vi "Splitting_without_Origin_Solution-1.vi"(6 "[IN] Crossconn\nection corrected":bool, 8 "error IN":errorcluster, 9 "[IN] # of Track with\nFirst Problem Point":i32, 10 "[IN] Index of First Pro\nblem Point Inside Track":i32, 11 "[IN] Still connected\ntracks in group":T2) -> (0 "error OUT":errorcluster, 3 "[OUT] Clusters for Re\nconstructed Tracks":T1, 4 "[OUT] Problem with 11 Point\nwithout Origin Resolved":bool)   [LabVIEW 2013]
doc: "Suprogram resolves the problem of splitting with no origin: \n- if further points don't merge again (assumption that they aren't equaul to \"101\" or \"111\") \n - then splitting points just loose their problem status and become origins for two different tracks"
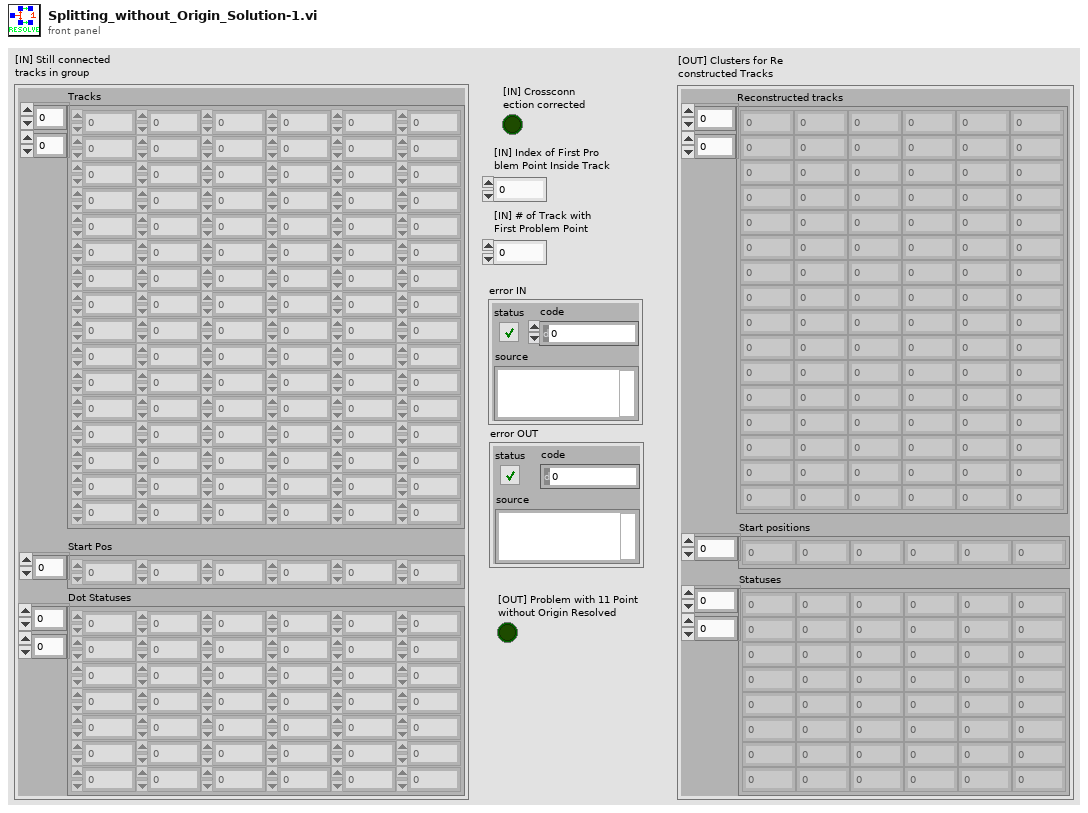
[diagram p1: front panel]
types:
  T1 = cluster{"Reconstructed tracks":dbl[][], "Start positions":i32[], "Statuses":i16[][]}
  T2 = cluster{"Tracks":dbl[][], "Start Pos":i32[], "Dot Statuses":i16[][]}
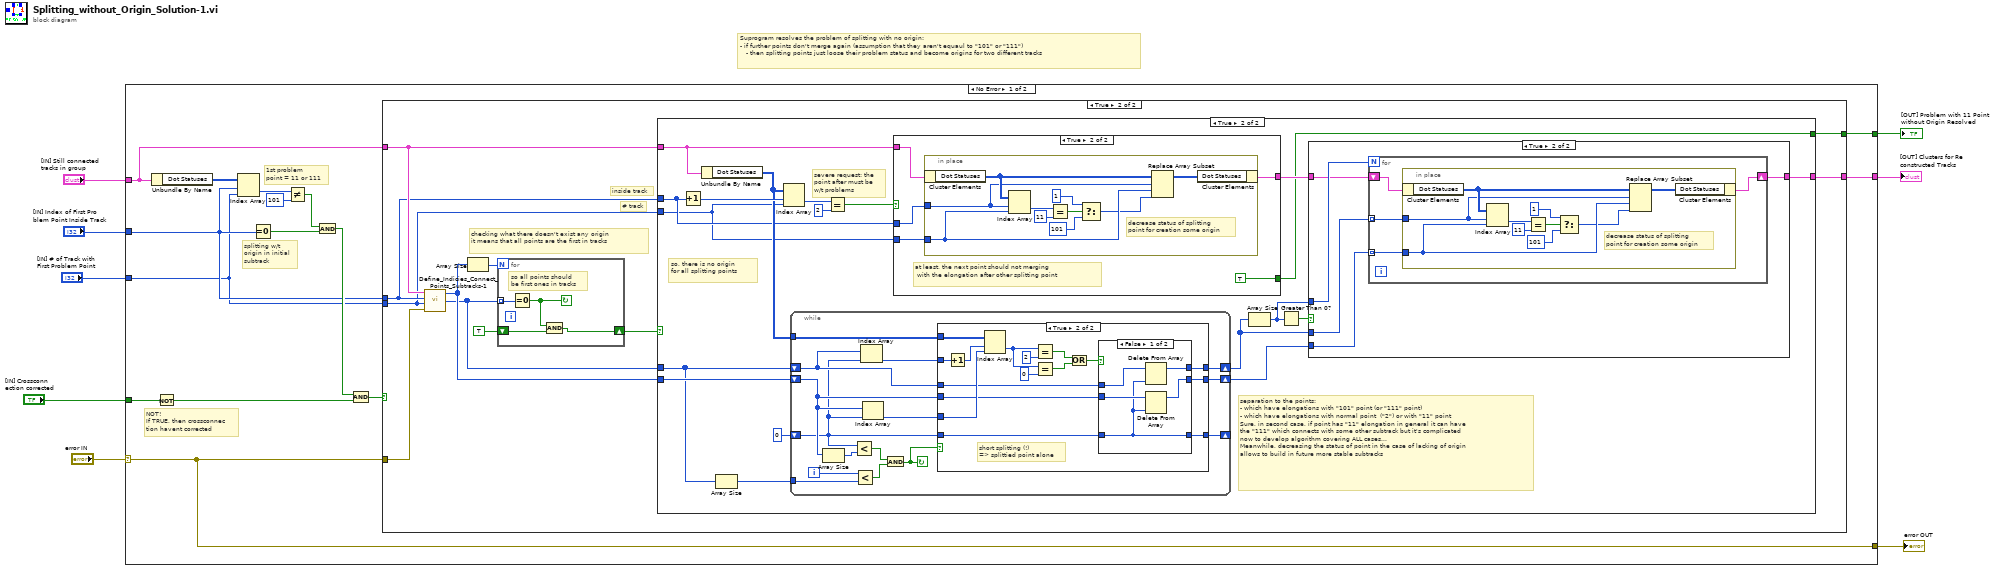
[diagram p0: block diagram]
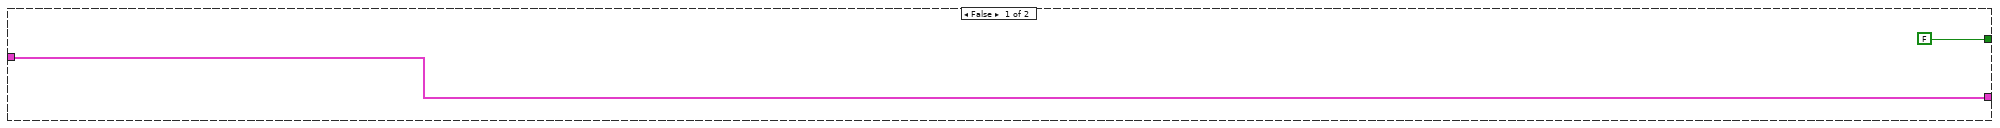
[diagram p2: hidden frame]
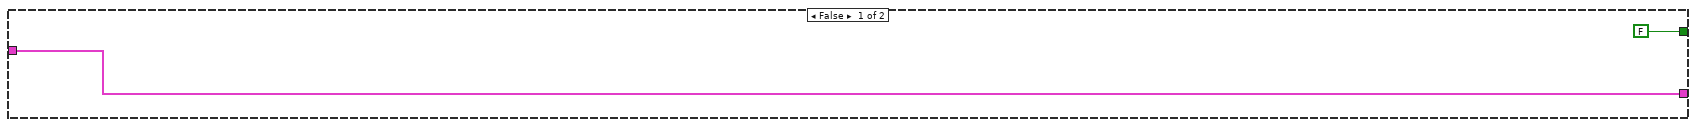
[diagram p3: hidden frame]
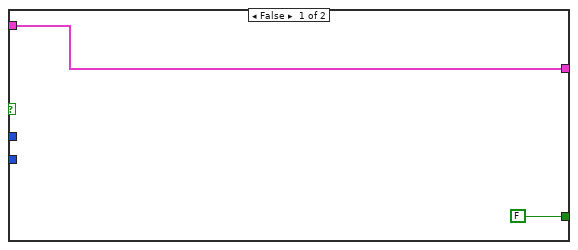
[diagram p5: hidden frame]
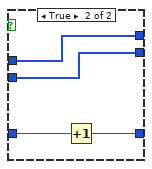
[diagram p7: hidden frame]
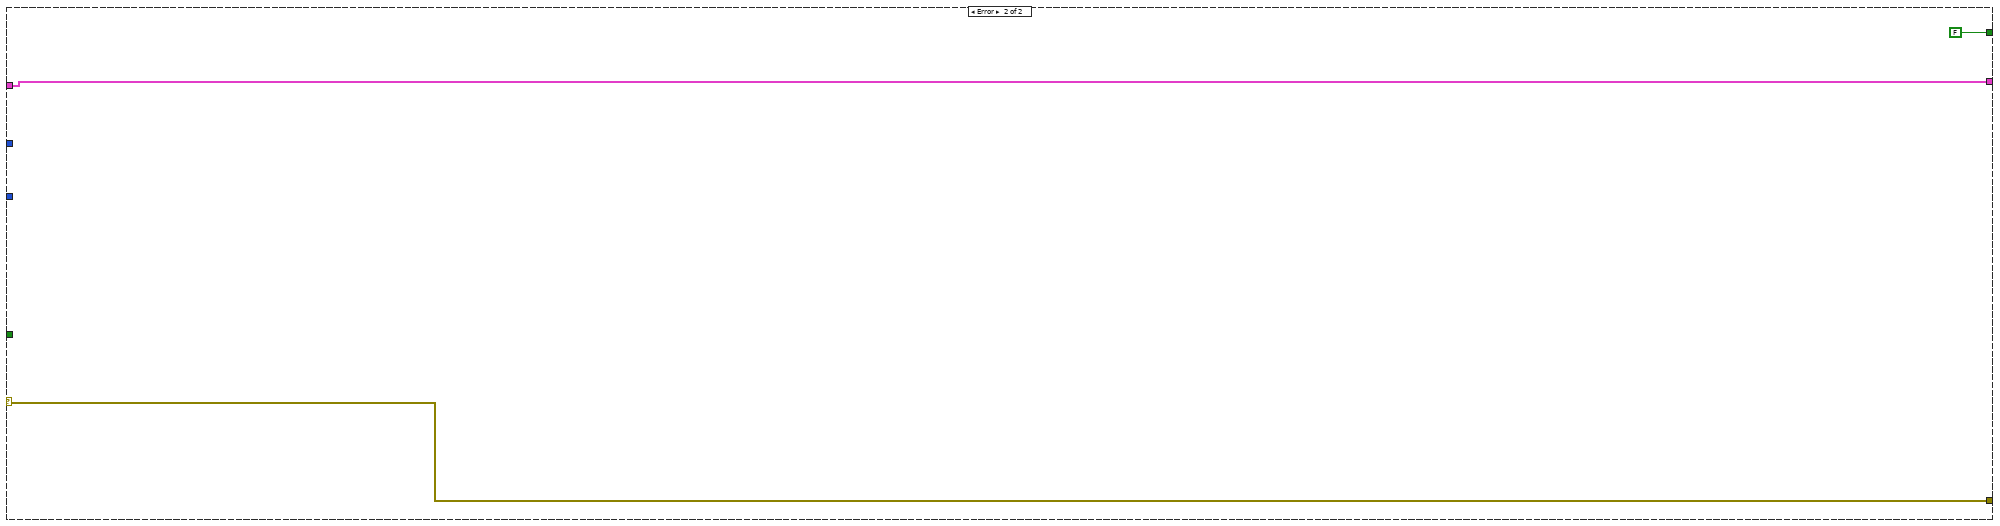
[diagram p8: hidden frame]
diagram:
  # "Suprogram resolves the problem of splitting with no origin: \n- if further points don't merge again (assumption that they aren't equaul to \"101\" or \"111\") \n   - then splitting points just loose their problem status and become origins for two different tracks"
  n1 = case shown="No Error" "error IN" {
    selector: "error IN" -> [w11 w144]
    tunnel: "[IN] Crossconn\nection corrected" -> [w23 _]
    tunnel: "[IN] Still connected\ntracks in group" -> [w15 w142]
    tunnel: "[IN] Index of First Pro\nblem Point Inside Track" -> [w14 _]
    tunnel: "[IN] # of Track with\nFirst Problem Point" -> [w13 _]
    tunnel: [w11 w144] -> w3
    tunnel: [w10 FALSE] -> w1
    tunnel: [w9 w142] -> w2
    frame No Error {
      # "splitting w/t \norigin in initial\nsubtrack"
      # "1st problem\npoint = 11 or 111"
      # "NOT! \nIf TRUE, then crossconnec\ntion havent corrected"
      n2 = Unbundle By Name(w15) -> ("Dot Statuses"=w12:i16[][])
      n3 = Not(x=w23) -> (.not. x?=w20:bool)
      n4 = Index Array(array=w12, index (row)=w14, index (col)=w13) -> (element=w22:i16)
      n5 = Equal To 0?(x=w14) -> (x = 0?=w17:bool)
      n6 = Not Equal?(x=w22, y=i16 101) -> (x != y?=w18:bool)
      n7 = And(x=w18, y=w17) -> (x .and. y?=w16:bool)
      n8 = And(x=w16, y=w20) -> (x .and. y?=w19:bool)
      n9 = case shown="True" w19 {
        tunnel: w11 -> [_ w36]
        tunnel: w15 -> [w24 w32]
        tunnel: w14 -> [_ w29]
        tunnel: w13 -> [_ w28]
        tunnel: [w24 w27] -> w9
        tunnel: [FALSE w26] -> w10
        frame False {
        }
        frame True {
          # "# track"
          # "inside track"
          # "checking what there doesn't exist any origin\nit means that all points are the first in tracks"
          n10 = call "Define_Indicies_Connect_Points_Subtracks-1.vi"("error IN"=w36, "[IN] Index of track with\n(problem displacement)"=w28, "[IN] Index of problem\ndisplacement inside track"=w29, "[IN] Track group"=w32) -> ("[OUT] Index of \nconnected dots\ninside the track"=w30:i32[], "[OUT] Index of connected\ntracks with problem dot"=w31:i32[])  [unwired: 1 out]
          n11 = Array Size(array=w31) -> (size(s)=w35:i32)
          n12 = for {
            N: w35 -> [_]
            tunnel: w30 -> [w141] mode=indexing
            shift-right: [w138] -> w33
            shift-left: TRUE -> [w140]
            stop <- w139 continue-if-true
            # "so all points should \nbe first ones in tracks"
            n13 = Equal To 0?(x=w141) -> (x = 0?=w139:bool)
            n14 = And(x=w139, y=w140) -> (x .and. y?=w138:bool)
          }
          n15 = case shown="True" w33 {
            tunnel: w32 -> [w37 w52]
            tunnel: w31 -> [_ w56]
            tunnel: w30 -> [_ w48]
            tunnel: w29 -> [_ w51]
            tunnel: w28 -> [_ w50]
            tunnel: [FALSE w41] -> w26
            tunnel: [w37 w40] -> w27
            frame False {
            }
            frame True {
              # "severe request: the \npoint after must be \nw/t problems"
              # "separation to the points: \n- which have elongations with \"101\" point (or \"111\" point)\n- which have elongations with normal point  (\"2\") or with \"11\" point\nSure, in second case, if point has \"11\" elongation in general it can have\nthe \"111\" which connects with some other subtrack but it's complicated\nnow to develop algorithm covering ALL cases...\nMeanwhile, decreasing the status of point in the case of lacking of origin\nallows to build in future more stable subtracks"
              # "so, there is no origin \nfor all splitting points"
              n16 = Increment(x=w51) -> (x+1=w57:i32)
              n17 = Unbundle By Name(w52) -> ("Dot Statuses"=w53:i16[][])
              n18 = Array Size(array=w48) -> (size(s)=w47:i32)
              n19 = Index Array(array=w53, index (row)=w57, index (col)=w50) -> (element=w54:i16)
              n20 = while {
                shift-right: [w96] -> w43
                shift-left: w48 -> [w100]
                shift-right: [w95] -> w42
                shift-left: w56 -> [w99]
                tunnel: w53 -> [w101]
                shift-right: [w97] -> _
                shift-left: 0 -> [w98]
                tunnel: w47 -> [w107]
                i -> [w108]
                stop <- w103 continue-if-true
                n21 = Array Size(array=w99) -> (size(s)=w109:i32)
                n22 = Less?(x=w98, y=w109) -> (x < y?=w106:bool)
                n23 = Less?(x=w108, y=w107) -> (x < y?=w105:bool)
                n24 = Index Array(array=w100, index=w98) -> (element=w102:i32)
                n25 = Index Array(array=w99, index=w98) -> (element=w104:i32)
                n26 = And(x=w106, y=w105) -> (x .and. y?=w103:bool)
                n27 = case shown="True" w103 {
                  tunnel: w104 -> [_ w125]
                  tunnel: w102 -> [_ w127]
                  tunnel: w101 -> [_ w128]
                  tunnel: w100 -> [w112 w123]
                  tunnel: w99 -> [w110 w122]
                  tunnel: w98 -> [w111 w121]
                  tunnel: [w111 w120] -> w97
                  tunnel: [w112 w119] -> w96
                  tunnel: [w110 w118] -> w95
                  frame False {
                  }
                  frame True {
                    # "short splitting (!)\n=> splittied point alone"
                    n28 = Increment(x=w127) -> (x+1=w126:i32)
                    n29 = Index Array(array=w128, index (row)=w126, index (col)=w125) -> (element=w117:i16)
                    n30 = Equal?(x=w117, y=i16 2) -> (x = y?=w113:bool)
                    n31 = Equal?(x=w117, y=i16 0) -> (x = y?=w114:bool)
                    n32 = Or(x=w113, y=w114) -> (x .or. y?=w115:bool)
                    n33 = case shown="False" w115 {
                      tunnel: w123 -> [w133 w135]
                      tunnel: w122 -> [w132 w134]
                      tunnel: w121 -> [w131 w137]
                      tunnel: [w131 w136] -> w120
                      tunnel: [w130 w135] -> w119
                      tunnel: [w129 w134] -> w118
                      frame False {
                        n34 = Delete From Array(array=w133, index=w131) -> (array with subset deleted=w130:i32[])  [unwired: 1 in, 1 out]
                        n35 = Delete From Array(array=w132, index=w131) -> (array with subset deleted=w129:i32[])  [unwired: 1 in, 1 out]
                      }
                      frame True {
                        n36 = Increment(x=w137) -> (x+1=w136:i32)
                      }
                    }
                  }
                }
              }
              n37 = Equal?(x=w54, y=i16 2) -> (x = y?=w39:bool)
              n38 = case shown="True" w39 {
                tunnel: w52 -> [w79 w84]
                tunnel: w51 -> [_ w83]
                tunnel: w50 -> [_ w82]
                tunnel: [w79 w81] -> w44
                tunnel: [FALSE TRUE] -> w41
                frame False {
                }
                frame True {
                  # "at least, the next point should not merging\n with the elongation after other splitting point"
                  n39 = in-place {
                    in-place-border: w83 -> [w91]
                    in-place-border: w82 -> [w87]
                    # "decrease status of splitting\npoint for creation some origin"
                    n40 = in-place-cluster #1(w84) -> ("Dot Statuses"=w94:i16[][])
                    n41 = Index Array(array=w94, index (row)=w91, index (col)=w87) -> (element=w93:i16)
                    n42 = Equal?(x=w93, y=i16 11) -> (x = y?=w90:bool)
                    n43 = Select(t=i16 1 ("y"), s=w90, f=i16 101 ("y")) -> (s? t:f=w86:i16)
                    n44 = Replace Array Subset(array=w94, new element=w86, index (row)=w91, index (col)=w87) -> (w85:i16[][])
                    n45 = in-place-cluster #1("Dot Statuses"=w85) -> (w81:T2)
                  }
                }
              }
              n46 = Array Size(array=w43) -> (size(s)=w45:i32)
              n47 = Greater Than 0?(x=w45) -> (x > 0?=w46:bool)
              n48 = case shown="True" w46 {
                tunnel: w45 -> [_ w63]
                tunnel: w44 -> [w58 w62]
                tunnel: w43 -> [_ w61]
                tunnel: w42 -> [_ w60]
                tunnel: [w58 w59] -> w40
                frame False {
                }
                frame True {
                  n49 = for {
                    N: w63 -> [_]
                    shift-right: [w66] -> w59
                    shift-left: w62 -> [w67]
                    tunnel: w61 -> [w65] mode=indexing
                    tunnel: w60 -> [w64] mode=indexing
                    n50 = in-place {
                      in-place-border: w65 -> [w74]
                      in-place-border: w64 -> [w70]
                      # "decrease status of splitting\npoint for creation some origin"
                      n51 = in-place-cluster #2(w67) -> ("Dot Statuses"=w77:i16[][])
                      n52 = Index Array(array=w77, index (row)=w74, index (col)=w70) -> (element=w76:i16)
                      n53 = Equal?(x=w76, y=i16 11) -> (x = y?=w73:bool)
                      n54 = Select(t=i16 1 ("y"), s=w73, f=i16 101 ("y")) -> (s? t:f=w69:i16)
                      n55 = Replace Array Subset(array=w77, new element=w69, index (row)=w74, index (col)=w70) -> (w68:i16[][])
                      n56 = in-place-cluster #2("Dot Statuses"=w68) -> (w66:T2)
                    }
                  }
                }
              }
            }
          }
        }
      }
    }
    frame Error {
    }
  }
  "[OUT] Clusters for Re\nconstructed Tracks" <- w2
  "error OUT" <- w3
  "[OUT] Problem with 11 Point\nwithout Origin Resolved" <- w1
